vi "Append Report Text (num).vi"(0 "report in":refnum<class "NI_Word.lvclass">, 1 "MS Office parameters":T1, 2 "format string (%.3f)":string="%.3f", 7 "text":dbl format="%.2f", 9 "append on new line? (F)":bool, 11 "error in (no error)":errorcluster) -> (4 "report out":refnum<class "NI_Word.lvclass">, 8 "start out (Word)":i32, 10 "end out (Word)":i32, 15 "error out":errorcluster)   [LabVIEW 2020, in "NI_Word.lvclass"]
doc: "Appends text to the selected report."
uses:
  <vilib>/Utility/NIReport.llb/Word/NI_Word.lvclass
  <vilib>/Utility/NIReport.llb/Word/NI_Word.lvclass/NI_Word.ctl
  <vilib>/addons/_office/NI_ReportGenerationToolkit.lvlib
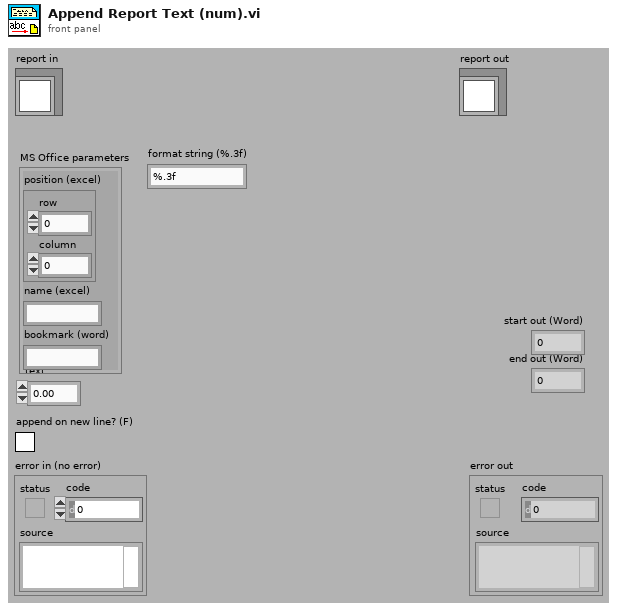
[diagram p1: front panel]
types:
  T1 = cluster{"position (excel)":cluster{"row":i32, "column":i32}, "name (excel)":string, "bookmark (word)":string}
  T2 = typedef "NI_ReportGenerationCore.lvlib/Report Data Members.ctl" = cluster{"font":T3, "from template?":bool}
  T3 = typedef "NI_ReportGenerationCore.lvlib/font.ctl" = cluster{"font name":string, "font size":dbl, "bold":u16, "italic":u16, "underline":u16, "strike through":u16, "font color":u32}
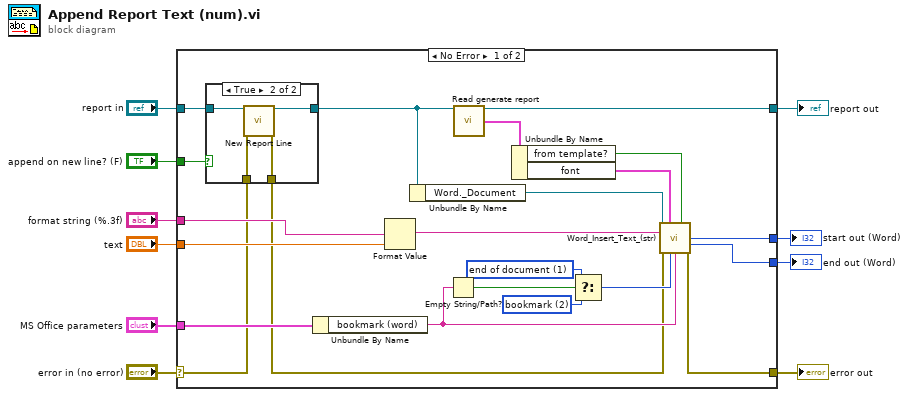
[diagram p0: block diagram]
diagram:
  n1 = case shown="No Error" "error in (no error)" {
    selector: "error in (no error)" -> [w17 w40]
    tunnel: [w20 w40] -> w9
    tunnel: [w14 w39] -> w7
    tunnel: "report in" -> [w32 w39]
    tunnel: "append on new line? (F)" -> [w31 _]
    tunnel: "MS Office parameters" -> [w23 _]
    tunnel: [w22 _] -> w4
    tunnel: [w21 _] -> w3
    tunnel: "text" -> [w19 _]
    tunnel: "format string (%.3f)" -> [w18 _]
    frame No Error {
      w24 = u16 2 items=["begining of document", "end of document", "bookmark", "custom"] ("Insertion point")
      w25 = u16 1 items=["begining of document", "end of document", "bookmark", "custom"] ("Insertion point")
      n2 = case shown="True" w31 {
        tunnel: w32 -> [w34 w38]
        tunnel: [w34 w37] -> w15
        tunnel: w17 -> [w33 w36]
        tunnel: [w33 w35] -> w16
        frame False {
        }
        frame True {
          n3 = call-dynamic "New Report Line.vi"("report in"=w38, "error in (no error)"=w36) -> ("report out"=w37:refnum<class "NI_Word.lvclass">, "error out"=w35:errorcluster)  [unwired: 12 in]
        }
      }
      n4 = Unbundle By Name(w23) -> ("bookmark (word)"=w27:string)
      n5 = Format Value(format string=w18, value (0)=w19) -> (output string=w30:string)  [unwired: 1 out]
      n6 = Unbundle By Name(w15) -> ("Word._Document"=w29:refnum<k7>)
      n7 = Empty String/Path?(string/path=w27) -> (empty?=w26:bool)
      n8 = call-dynamic "Read generate report.vi"("report in"=w15) -> ("report out"=w14:refnum<class "NI_Word.lvclass">, "generate report"=w11:T2)  [unwired: 12 in, 1 out]
      n9 = Unbundle By Name(w11) -> ("from template?"=w13:bool, "font"=w12:T3)
      n10 = Select(t=w25, s=w26, f=w24) -> (s? t:f=w28:u16)
      n11 = call <vilib>:"Word_Insert_Text_(str).vi"("Word._Document"=w29, "font"=w12, "from template?"=w13, "Text"=w30, "Error in (no error)"=w16, "Insertion point"=w28, "Bookmark name"=w27) -> ("Start out"=w22:i32, "End out"=w21:i32, "Error out"=w20:errorcluster)  [unwired: 3 in, 3 out]
    }
    frame Error {
    }
  }
  "error out" <- w9
  "report out" <- w7
  "start out (Word)" <- w4
  "end out (Word)" <- w3
